vi "Open or Closed Loop.vi"(0 "Mode":enum16{"Init", "Settings", "Run"}(ring)=enum."Run", 1 "VSig":refnum<vi>, 2 "PresSig":refnum<vi>, 5 "VPID":dbl, 9 "PresPID":dbl, 11 "VDirect":dbl, 12 "DirectV?":bool, 13 "PresDirect":dbl, 14 "DirectPres?":bool) -> (6 "VSig":dbl, 10 "PresSig":dbl)   [LabVIEW 2019]
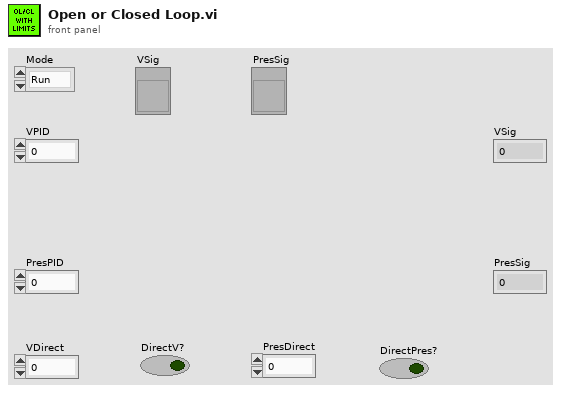
[diagram p1: front panel]
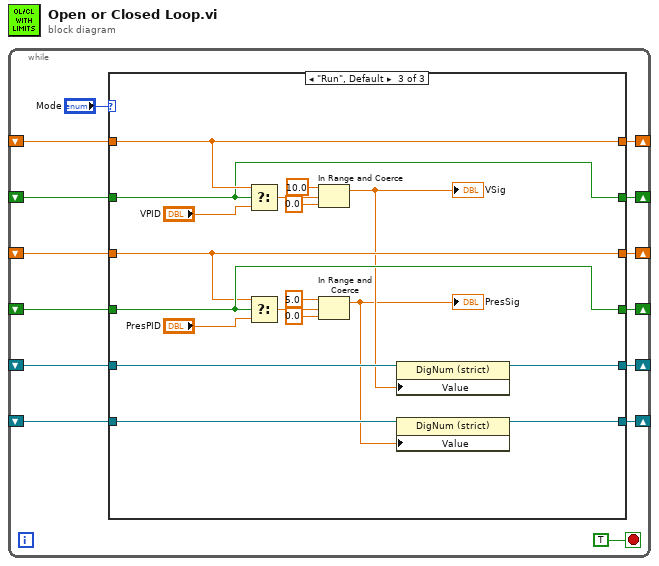
[diagram p0: block diagram]
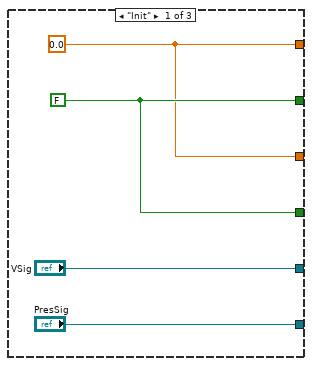
[diagram p2: hidden frame]
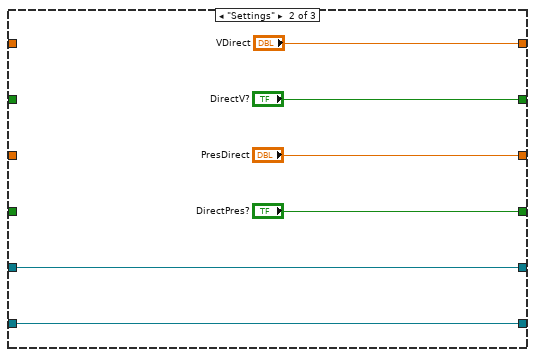
[diagram p3: hidden frame]
diagram:
  n1 = while {
    shift-right: [w7] -> _
    shift-left: _ -> [w1]
    shift-right: [w8] -> _
    shift-left: _ -> [w2]
    shift-right: [w9] -> _
    shift-left: _ -> [w3]
    shift-right: [w10] -> _
    shift-left: _ -> [w4]
    shift-right: [w11] -> _
    shift-left: _ -> [w5]
    shift-right: [w12] -> _
    shift-left: _ -> [w6]
    stop <- TRUE stop-if-true
    n2 = case shown="\"Run\", Default" "Mode" {
      tunnel: [w15 "VDirect" w34] -> w12
      tunnel: [w16 "DirectV?" w33] -> w11
      tunnel: [w15 "PresDirect" w31] -> w10
      tunnel: [w16 "DirectPres?" w32] -> w9
      tunnel: ["VSig" w24 w29] -> w8
      tunnel: ["PresSig" w23 w28] -> w7
      tunnel: w6 -> [_ _ w34]
      tunnel: w5 -> [_ _ w33]
      tunnel: w4 -> [_ _ w31]
      tunnel: w3 -> [_ _ w32]
      tunnel: w2 -> [_ w24 w30]
      tunnel: w1 -> [_ w23 w27]
      frame "Init" {
        w16 = FALSE ("DirectV?")
        w15 = 0.0 ("VDirect")
      }
      frame "Settings" {
      }
      frame "Run", Default {
        n3 = Select(t=w34, s=w33, f="VPID") -> (s? t:f=w39:dbl)
        n4 = Select(t=w31, s=w32, f="PresPID") -> (s? t:f=w38:dbl)
        n5 = In Range and Coerce(upper limit=10.0, x=w39, lower limit=0.0) -> (coerced(x)=w26:dbl)  [unwired: 1 out]
        "VSig" <- w26
        n6 = In Range and Coerce(upper limit=5.0, x=w38, lower limit=0.0) -> (coerced(x)=w25:dbl)  [unwired: 1 out]
        "PresSig" <- w25
        n7 = property class="DigNum (strict)"(reference=w30, "Value"=w26) -> (reference out=w29:refnum<vi>)  [unwired: 1 in, 1 out]
        n8 = property class="DigNum (strict)"(reference=w27, "Value"=w25) -> (reference out=w28:refnum<vi>)  [unwired: 1 in, 1 out]
      }
    }
  }
